vi "Two Shimmer.vi"() -> ()   [LabVIEW 2025]
uses:
  C:/Github/Shimmer-Labview/ShimmerLV_Test/ShimmerLVWrapper.dll
  ShimmerLVWrapper.dll
panel:
  out "Waveform Chart 2":cluster{dbl, dbl, dbl}(graph)
  out "Waveform Chart":cluster{dbl, dbl, dbl}(graph)
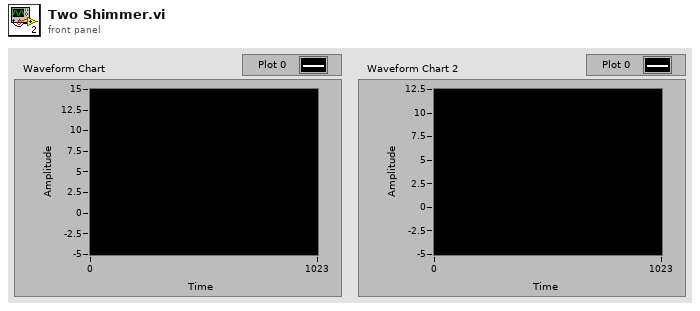
[diagram p1: front panel]
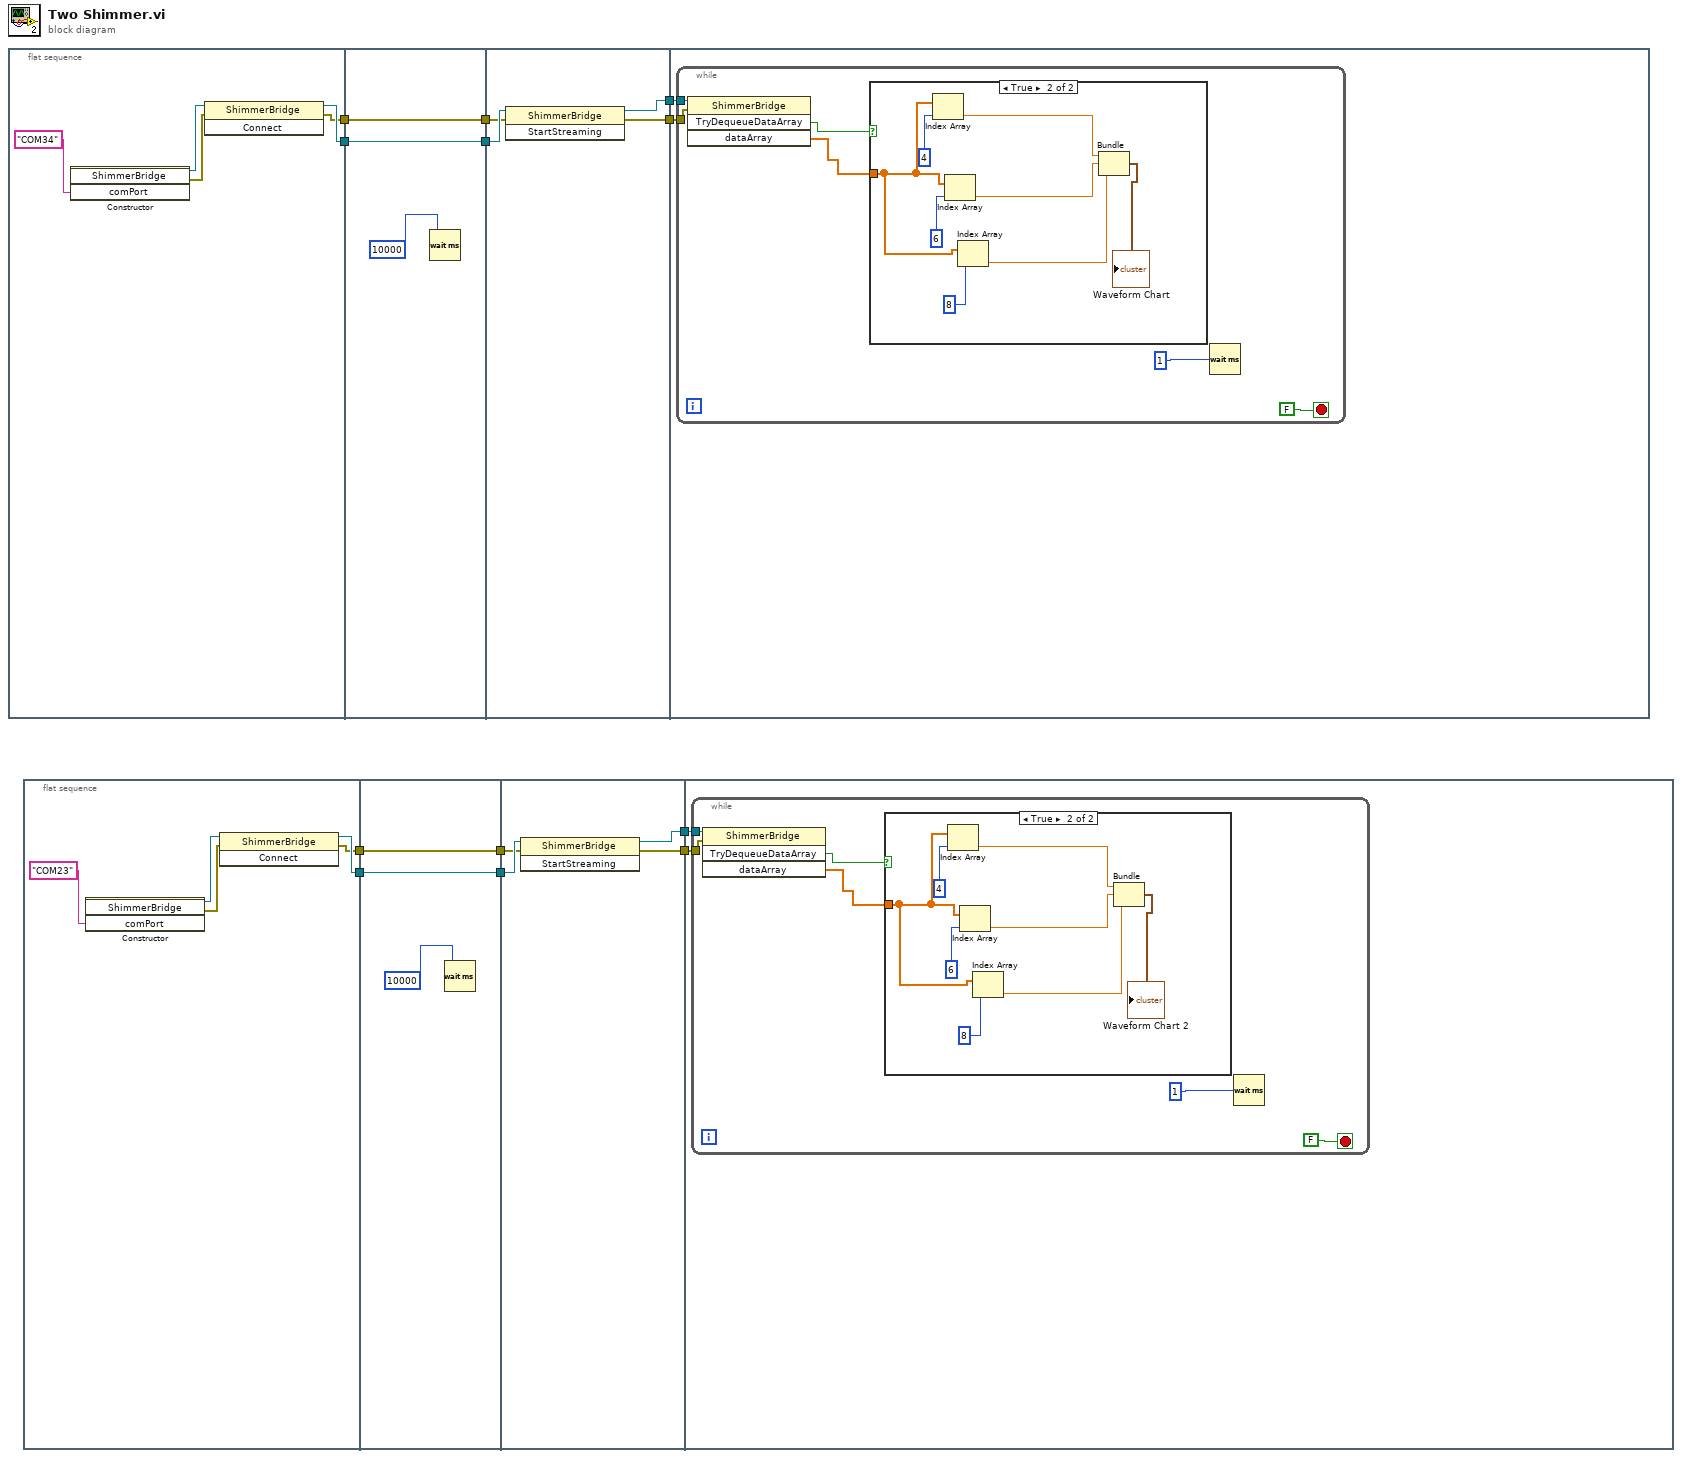
[diagram p0: block diagram]
diagram:
  n1 = flat-sequence {
    tunnel: [w14] -> w12
    tunnel: [w13] -> w5
    tunnel: w12 -> [w19]
    tunnel: [w19] -> w11
    tunnel: [w18] -> w6
    tunnel: w5 -> [w18]
    tunnel: w11 -> [w24]
    tunnel: [w23] -> w10
    tunnel: w6 -> [w22]
    tunnel: [w21] -> w4
    tunnel: w10 -> [w26]
    tunnel: w4 -> [w25]
    frame #0 {
      n2 = constructor class="ShimmerBridge"("comPort"="COM34") -> (reference out=w16:refnum<k24>, error out=w15:errorcluster)  [unwired: 3 in, 2 out]
      n3 = invoke class="ShimmerBridge" method="Connect"(reference=w16, error in=w15) -> (reference out=w14:refnum<k24>, error out=w13:errorcluster)  [unwired: 1 in, 1 out]
    }
    frame #1 {
      n4 = Wait (ms)(milliseconds to wait=u32 10000 ("millisecond timer value")) -> ()  [unwired: 1 out]
    }
    frame #2 {
      n5 = invoke class="ShimmerBridge" method="StartStreaming"(reference=w24, error in=w22) -> (reference out=w23:refnum<k24>, error out=w21:errorcluster)  [unwired: 1 in, 1 out]
    }
    frame #3 {
      n6 = while {
        tunnel: w26 -> [w30]
        tunnel: w25 -> [w27]
        stop <- FALSE stop-if-true
        n7 = invoke class="ShimmerBridge" method="TryDequeueDataArray"(reference=w30, error in=w27) -> ("TryDequeueDataArray"=w29:bool, "dataArray"=w28:dbl[])  [unwired: 2 in, 2 out]
        n8 = case shown="True" w29 {
          tunnel: w28 -> [_ w37]
          frame False {
          }
          frame True {
            n9 = Index Array(array=w37, index=4) -> (element=w36:dbl)
            n10 = Index Array(array=w37, index=6) -> (element=w35:dbl)
            n11 = Index Array(array=w37, index=8) -> (element=w34:dbl)
            n12 = Bundle(w36, w35, w34) -> (→"Waveform Chart":cluster{dbl, dbl, dbl})  [unwired: 1 in]
          }
        }
        n13 = Wait (ms)(milliseconds to wait=u32 1) -> ()  [unwired: 1 out]
      }
    }
  }
  n14 = flat-sequence {
    tunnel: [w42] -> w9
    tunnel: [w41] -> w2
    tunnel: w9 -> [w47]
    tunnel: [w47] -> w8
    tunnel: [w46] -> w3
    tunnel: w2 -> [w46]
    tunnel: w8 -> [w52]
    tunnel: [w51] -> w7
    tunnel: w3 -> [w50]
    tunnel: [w49] -> w1
    tunnel: w7 -> [w54]
    tunnel: w1 -> [w53]
    frame #0 {
      n15 = constructor class="ShimmerBridge"("comPort"="COM23") -> (reference out=w44:refnum<k24>, error out=w43:errorcluster)  [unwired: 3 in, 2 out]
      n16 = invoke class="ShimmerBridge" method="Connect"(reference=w44, error in=w43) -> (reference out=w42:refnum<k24>, error out=w41:errorcluster)  [unwired: 1 in, 1 out]
    }
    frame #1 {
      n17 = Wait (ms)(milliseconds to wait=u32 10000 ("millisecond timer value")) -> ()  [unwired: 1 out]
    }
    frame #2 {
      n18 = invoke class="ShimmerBridge" method="StartStreaming"(reference=w52, error in=w50) -> (reference out=w51:refnum<k24>, error out=w49:errorcluster)  [unwired: 1 in, 1 out]
    }
    frame #3 {
      n19 = while {
        tunnel: w54 -> [w58]
        tunnel: w53 -> [w55]
        stop <- FALSE stop-if-true
        n20 = invoke class="ShimmerBridge" method="TryDequeueDataArray"(reference=w58, error in=w55) -> ("TryDequeueDataArray"=w57:bool, "dataArray"=w56:dbl[])  [unwired: 2 in, 2 out]
        n21 = case shown="True" w57 {
          tunnel: w56 -> [_ w65]
          frame False {
          }
          frame True {
            n22 = Index Array(array=w65, index=4) -> (element=w64:dbl)
            n23 = Index Array(array=w65, index=6) -> (element=w63:dbl)
            n24 = Index Array(array=w65, index=8) -> (element=w62:dbl)
            n25 = Bundle(w64, w63, w62) -> (→"Waveform Chart 2":cluster{dbl, dbl, dbl})  [unwired: 1 in]
          }
        }
        n26 = Wait (ms)(milliseconds to wait=u32 1) -> ()  [unwired: 1 out]
      }
    }
  }
